vi "Get_Build.vi"(8 "error in (no error)":errorcluster, 11 "IB_Source_Build in":refnum<class "IB_Source_Build.lvclass">) -> (0 "error out":errorcluster, 2 "data":cluster{"Dependencies":T1[]}, 3 "IB_Source_Build out":refnum<class "IB_Source_Build.lvclass">)   [LabVIEW 2020, in "IB_Source_Build.lvclass"]
uses:
  <vilib>/AppBuilder/IB_Classes/Source/Container/Build/IB_Source_Build.lvclass
  <vilib>/AppBuilder/AB_Dependency.ctl
  <vilib>/Utility/lvfile.llb/LVFileType.ctl
  <vilib>/AppBuilder/IB_Classes/Source/Container/Build/IB_Source_Build.lvclass/IB_Source_Build.ctl
  <vilib>/Utility/lvfile.llb/NI_FileType.lvlib
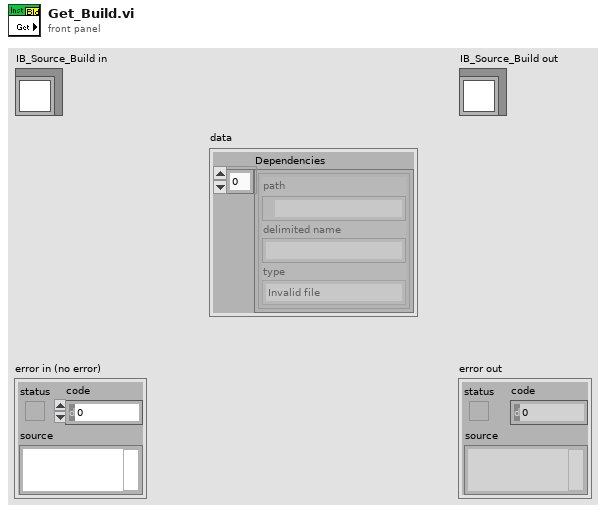
[diagram p1: front panel]
types:
  T1 = typedef "AB_Dependency.ctl" = cluster{"path":path, "delimited name":string, "type":T2}
  T2 = typedef "NI_FileType.lvlib/LVFileType.ctl" = enum32{"Invalid file", "Unknown type", "Instrument", "Control", "Polymorphic VI", "Project", "Library", "LVClass", "XControl", "XNode", "Shared library", ".NET assembly", "ActiveX interface", "CIN", "Run-time menu", "Palette menu", "Help file", "LLB", "XNode Edit Dependency", "Class Private Data Control", "Statechart", "MathScript .m file", "Ladder Diagram", "LVLibp", "XNode Build Dependency"}
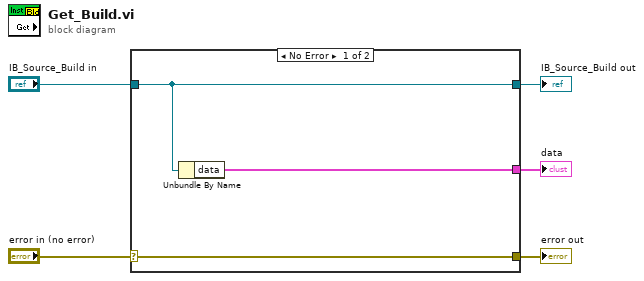
[diagram p0: block diagram]
diagram:
  n1 = case shown="No Error" "error in (no error)" {
    selector: "error in (no error)" -> [w8 w9]
    tunnel: [w8 w9] -> w4
    tunnel: [w7 w10] -> w2
    tunnel: "IB_Source_Build in" -> [w7 w10]
    tunnel: [w6 _] -> w1
    frame No Error {
      n2 = Unbundle By Name(w7) -> ("data"=w6:cluster{"Dependencies":T1[]})
    }
    frame Error {
    }
  }
  "error out" <- w4
  "IB_Source_Build out" <- w2
  "data" <- w1
